vi "Test subpanel.vi"() -> ()   [LabVIEW 2021]
uses:
  <vilib>/Utility/LVLibp/NI_PackedLibraryUtility.lvlib
panel:
  out "error out 4":errorcluster
  out "paths":path[](array[path])
  out "error out":errorcluster
  out "data out":string
  in  "stop":bool
  out "error out 3":errorcluster={"status"=TRUE, "code"=56, "source"="UDP Read in Test UDP launcher.vi"}
  out "error out 2":errorcluster
  out "qualified names":string[](array[string])=["CIFTemplatePlugin.lvlibp:Energize.vi", "CIFTemplatePlugin.lvlibp:Launch.vi"]
  in  "Linux":path=path "/home/lvuser/natinst/bin/CIFTemplatePlugin.lvlibp"
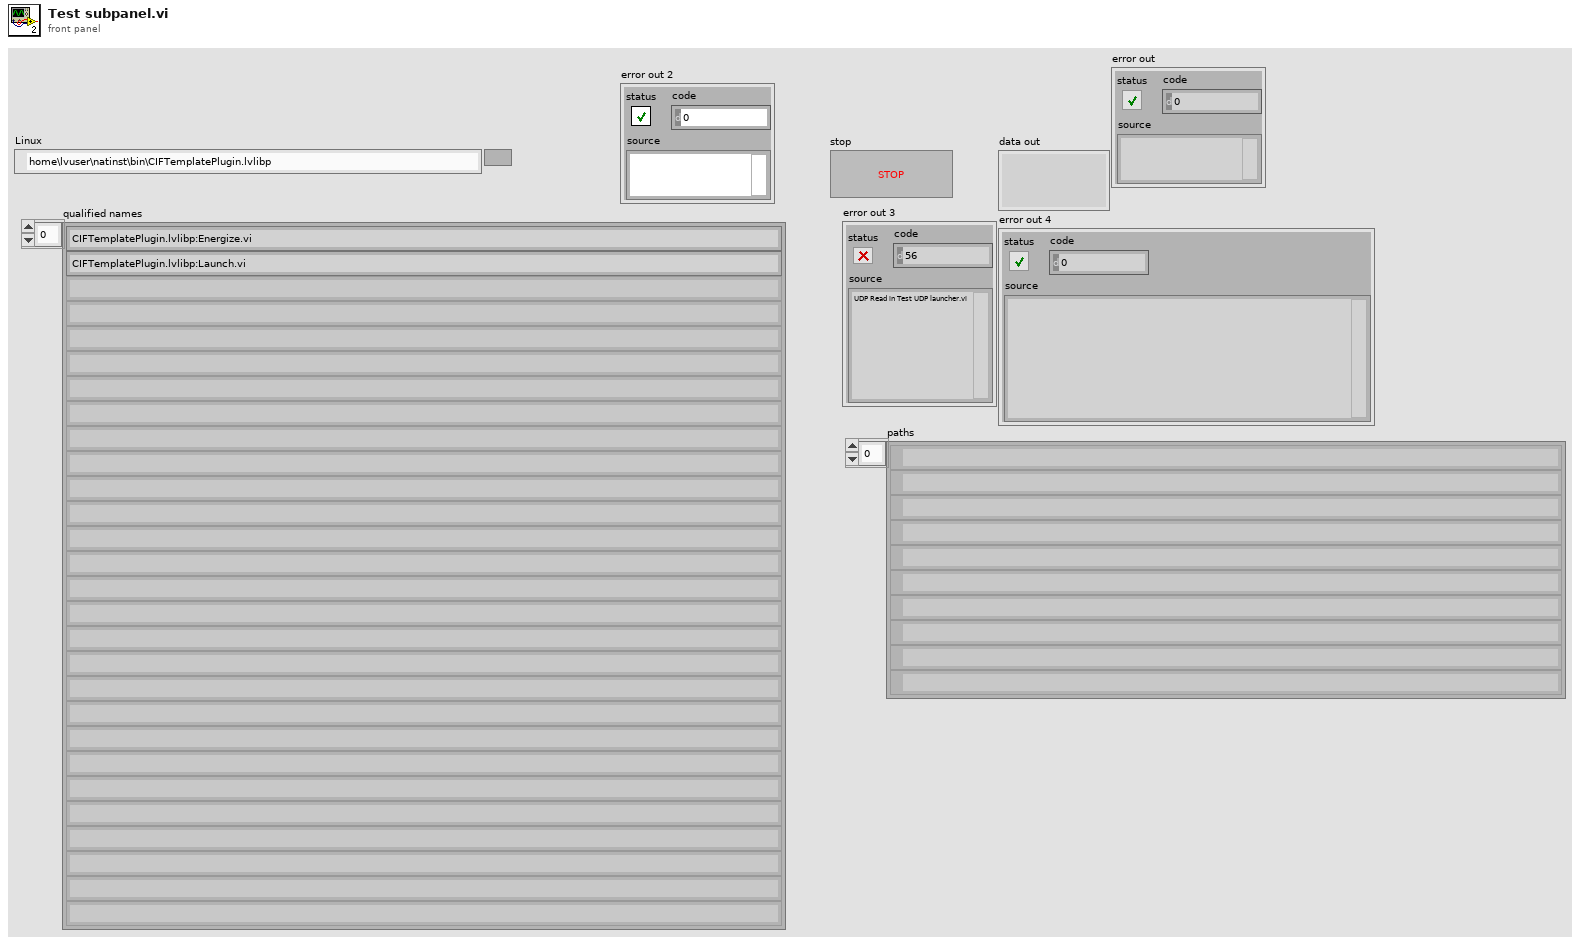
[diagram p1: front panel]
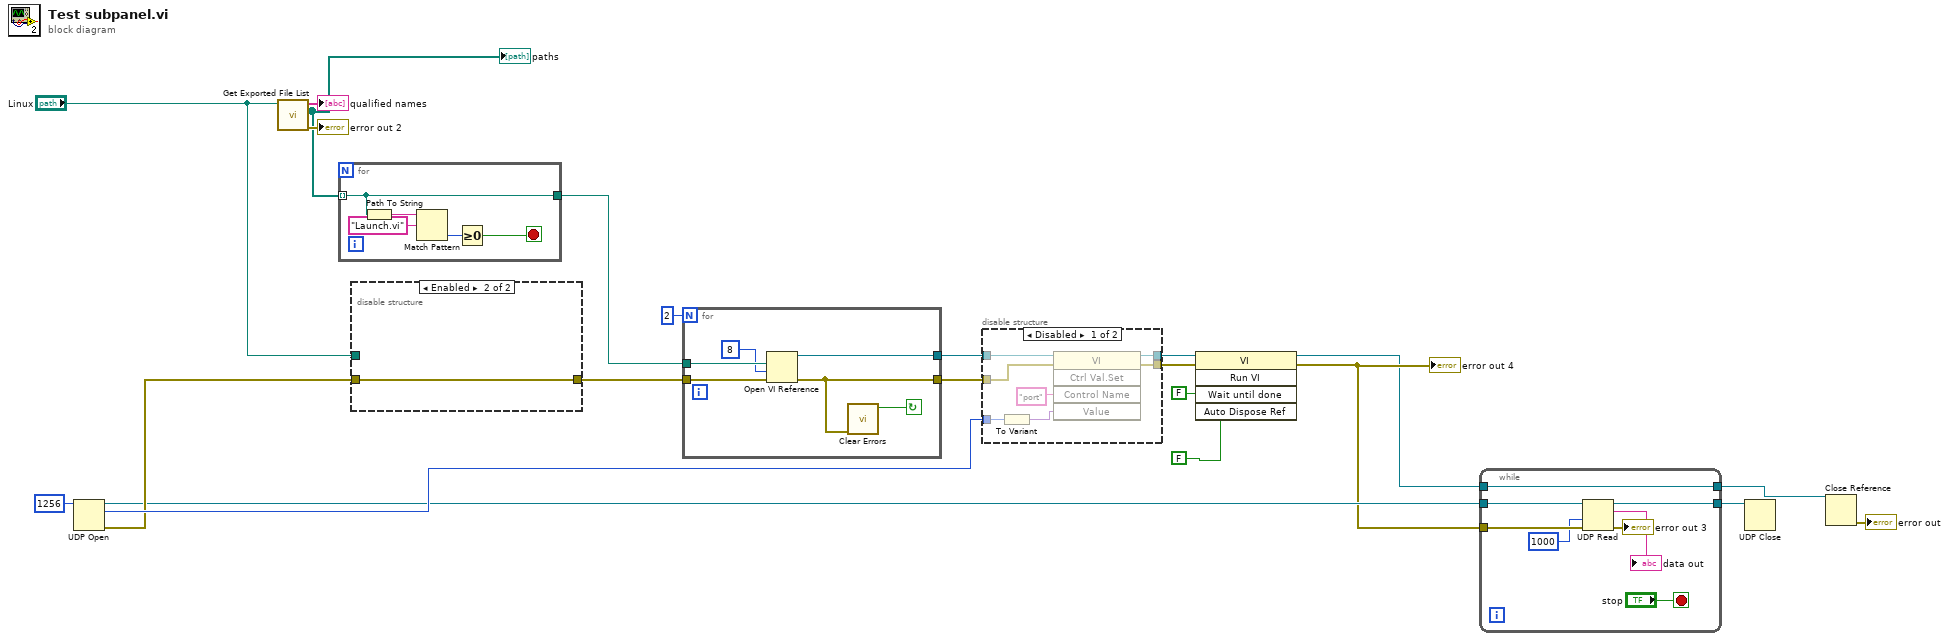
[diagram p0: block diagram]
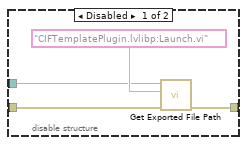
[diagram p2: hidden frame]
diagram:
  n1 = UDP Open(11:u16 1256 ("port")) -> (port=w17:refnum<k16>, 0:w18:errorcluster, 2:w19:u16)  [unwired: 4 in]
  n2 = call <vilib>:"Get Exported File List.vi"("packed library path"="Linux") -> ("error out"=→"error out 2":errorcluster, "paths"=w2:path[], "qualified names"=→"qualified names":string[])  [unwired: 8 in]
  "paths" <- w2
  n3 = for {
    tunnel: w2 -> [w23] mode=indexing
    tunnel: [w23] -> w1
    stop <- w24 stop-if-true
    n4 = Path To String(path=w23) -> (string=w27:string)
    n5 = Match Pattern(string=w27, regular expression="Launch.vi") -> (offset past match=w25:i32)  [unwired: 1 in, 3 out]
    n6 = Greater Or Equal To 0?(x=w25) -> (x >= 0?=w24:bool)
  }
  n7 = disable-structure shown="Enabled" {
    disable-tunnel: w18 -> [w31 w32]
    disable-tunnel: [w29 w32] -> w13
    disable-tunnel: "Linux" -> [w28 _]
    frame Disabled {
      n8 = call <vilib>:"Get Exported File Path.vi"("error in (no error)"=w31, "qualified name"="CIFTemplatePlugin.lvlibp:Launch.vi", "packed library path"=w28) -> ("error out"=w29:errorcluster)  [unwired: 7 in, 1 out]
    }
    frame Enabled {
    }
  }
  n9 = for {
    N: 2 -> [_]
    tunnel: w1 -> [w37]
    tunnel: [w36] -> w7
    tunnel: w13 -> [w38]
    tunnel: [w34] -> w14
    stop <- w33 continue-if-true
    n10 = Open VI Reference(vi path=w37, options=8, error in (no error)=w38) -> (vi reference=w36:refnum<vi>, error out=w34:errorcluster)  [unwired: 3 in]
    n11 = call <vilib>:"Clear Errors.vi"("error in (no error)"=w34) -> ("specific error cleared?"=w33:bool)  [unwired: 5 in, 1 out]
  }
  n12 = disable-structure shown="Disabled" {
    disable-tunnel: w19 -> [w45 _]
    disable-tunnel: [w42 w46] -> w8
    disable-tunnel: [w41 w47] -> w9
    disable-tunnel: w14 -> [w40 w46]
    disable-tunnel: w7 -> [w39 w47]
    frame Disabled {
      n13 = To Variant(anything=w45) -> (Variant=w44:variant)
      n14 = invoke class="VI" method="Ctrl Val.Set"(reference=w39, error in=w40, "Control Name"="port", "Value"=w44) -> (reference out=w41:refnum<vi>, error out=w42:errorcluster)  [unwired: 1 in, 3 out]
    }
    frame Enabled {
    }
  }
  n15 = invoke class="VI" method="Run VI"(reference=w9, error in=w8, "Wait until done"=FALSE ("Wait Until Done"), "Auto Dispose Ref"=FALSE ("Auto Dispose Reference")) -> (reference out=w6:refnum<vi>, error out=w10:errorcluster)  [unwired: 1 in, 3 out]
  "error out 4" <- w10
  n16 = while {
    tunnel: w17 -> [w55]
    tunnel: w10 -> [w54]
    tunnel: [w50] -> w12
    tunnel: w6 -> [w48]
    tunnel: [w48] -> w5
    stop <- "stop" stop-if-true
    n17 = UDP Read(connection ID=w55, timeout ms (25000)=1000, 8:w54) -> (data out=→"data out":string, error out=→"error out 3":errorcluster, 3:w50:refnum<k16>)  [unwired: 1 in, 2 out]
  }
  n18 = UDP Close(connection ID=w12) -> ()  [unwired: 1 in, 2 out]
  n19 = Close Reference(reference=w5) -> (error out=→"error out":errorcluster)  [unwired: 1 in]
